vi "SerialCommunication.vi"() -> ()   [LabVIEW 2011]
uses:
  <vilib>/FPGAPlugInAG/sbRIO-9636/niLvFpga_Open_sbRIO-9636.vi
  <vilib>/rvi/interface/common/dynamic/niFpgaDynamicAddResources.vi
  <vilib>/Utility/error.llb/Error Cluster From Error Code.vi
  <vilib>/rvi/errors/niLvFpgaAdjustHostInterfaceError.vi
  <vilib>/FPGAPlugInAG/Dynamic/niLvFpga_Run_Dynamic.vi
  <vilib>/FPGAPlugInAG/Dynamic/niLvFpga_Close_Dynamic.vi
  <vilib>/rvi/interface/nirviOpenFPGA/nirviOpenFPGA.xnode
  FPGA Bitfiles/TreadmillControl_FPGATarget_Exercise2_CF30559D.lvbitx
  FPGA/FPGA.vi
  <vilib>/rvi/interface/nirviReadWriteControl/nirviReadWriteControl.xnode
  <vilib>/rvi/interface/nirviMethod/nirviMethod.xnode
  <vilib>/rvi/interface/nirviCloseFPGA/nirviCloseFPGA.xnode
  NiFpgaLv.dll
  <vilib>/rvi/interface/Simulation/niFpgaSimulationCallBeginRW.vi
  <vilib>/FPGAPlugInAG/Dynamic/niLvFpga_ReadFifo_Dynamic.vi
  <vilib>/rvi/errors/niLvFpgaMergeErrorWithErrorCode.vi
panel:
  out "Elements Remaining":u32
  out "sum":u8
  in  "baud rate":u32=2500000
  out "PacketOut":u8[](array[numeric]) format="%02x"
  in  "Vl":i16
  in  "Vr":i16
  in  "Kff":u16
  in  "Kaw":u16
  in  "Kd":u16
  in  "Ki":u16
  in  "Kp":u16
  in  "PacketType":T1(ring)
  in  "Decimation":i32
  in  "EnableLog":bool
  in  "Right":u16 format="%x"
  in  "Left":u16 format="%x"
  out "Valid":bool
  out "ReadPacket":u8[](array[numeric]) format="%x"
  in  "Write":bool
  in  "Stop":bool
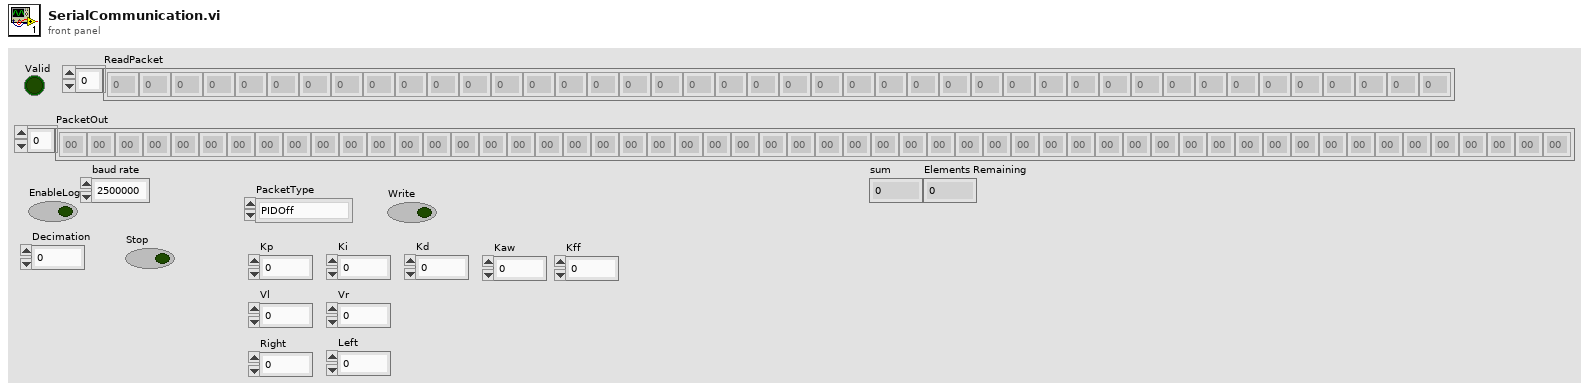
[diagram p1: front panel]
types:
  T1 = enum16{"PIDOff", "PIDOn", "PIDSetProfile", "PIDSetGains", "ThrustOpenLoop"}
  T2 = enum16{"open", "replace", "create", "open or create", "replace or create", "replace or create with confirmation"}
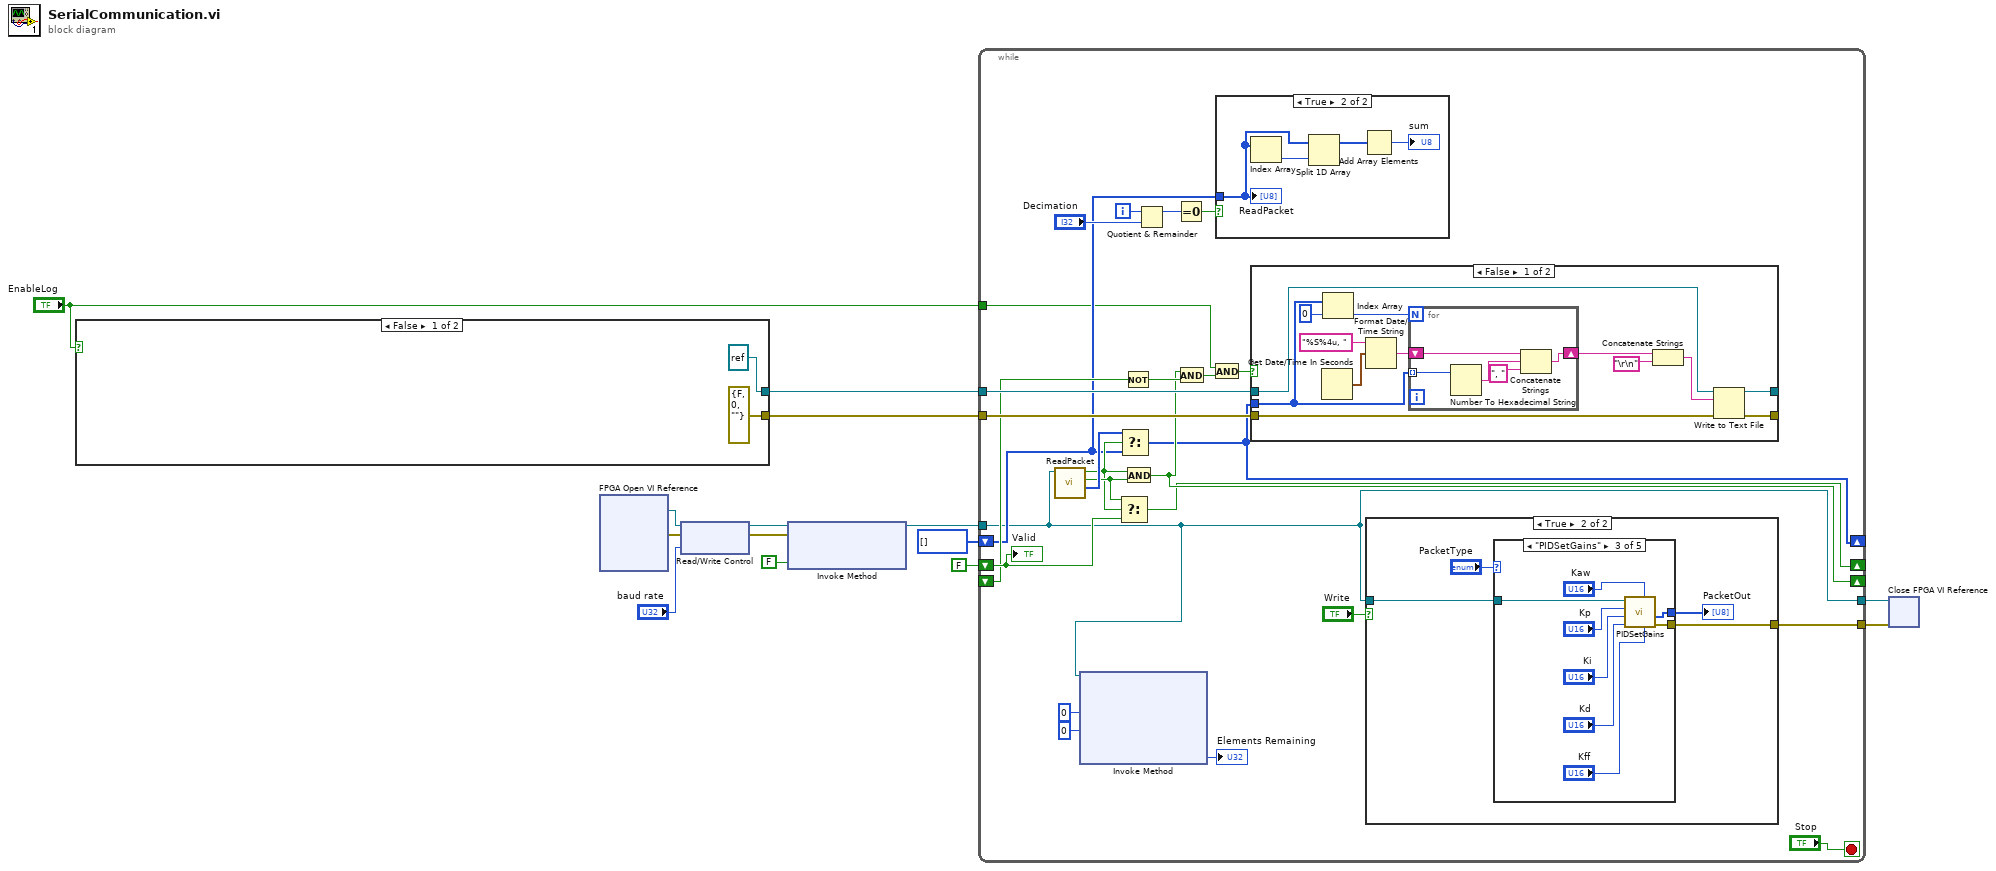
[diagram p0: block diagram]
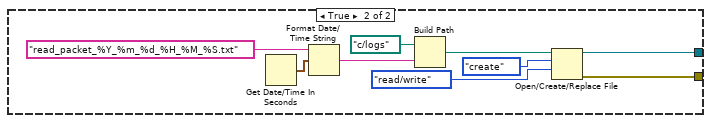
[diagram p2: hidden frame]
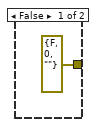
[diagram p5: hidden frame]
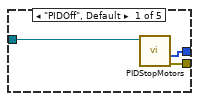
[diagram p6: hidden frame]
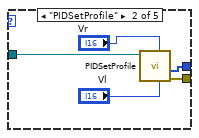
[diagram p7: hidden frame]
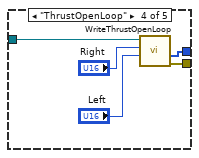
[diagram p8: hidden frame]
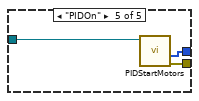
[diagram p9: hidden frame]
diagram:
  n1 = case shown="False" "EnableLog" {
    tunnel: [refnum<file> refnum ("refnum out") w18] -> w9
    tunnel: [errorcluster {"status"=FALSE, "code"=0, "source"=""} ("error out") w17] -> w8
    frame False {
    }
    frame True {
      n2 = Get Date/Time In Seconds() -> (seconds since 1Jan1904=w23:timestamp)
      n3 = Format Date/Time String(time format string (%c)="read_packet_%Y_%m_%d_%H_%M_%S.txt", seconds (now)=w23) -> (date/time string=w20:string)  [unwired: 1 in]
      n4 = Build Path(base path=path "c:/logs", name or relative path=w20) -> (appended path=w19:path)
      n5 = Open/Create/Replace File(file path (use dialog)=w19, operation (0:open)=T2."create", access (0:read/write)=enum16{"read/write", "read-only", "write-only"}."read/write") -> (refnum out=w18:refnum<file>, error out=w17:errorcluster)  [unwired: 3 in, 1 out]
    }
  }
  n6 = xnode "FPGA Open VI Reference"() -> ("FPGA VI Reference Out"=w5:refnum<k20>, "error out"=w3:errorcluster)  [unwired: 2 in]
  n7 = xnode "Read/Write Control"("FPGA VI Reference In"=w5, "error in"=w3, "baud rate"="baud rate") -> ("FPGA VI Reference Out"=w2:refnum<k20>, "error out"=w1:errorcluster)
  n8 = xnode "Invoke Method"("FPGA VI Reference In"=w2, "error in"=w1, "Wait Until Done (F)"=FALSE) -> ("FPGA VI Reference Out"=w6:refnum<k20>)  [unwired: 1 out]
  n9 = while {
    tunnel: w6 -> [w29]
    tunnel: [w50] -> w13
    tunnel: [w29] -> w12
    shift-right: [w37] -> _
    shift-left: u8[] [] ("ReadPacket") -> [w31]
    shift-right: [w36] -> _
    shift-left: FALSE ("Valid") -> [w47]
    tunnel: w9 -> [w45]
    tunnel: w8 -> [w44]
    shift-right: [w41] -> _
    shift-left: _ -> [w43]
    tunnel: "EnableLog" -> [w30]
    i -> [w35]
    stop <- "Stop" stop-if-true
    n10 = call "ReadPacket.vi"("Refnum in"=w29) -> ("ReadPacket"=w48:u8[], "Valid"=w46:bool, "Complete"=w40:bool)  [unwired: 8 in]
    n11 = xnode "Invoke Method"("FPGA VI Reference In"=w29, "Number of Elements"=u32 0, "Timeout (ms)"=0) -> ("Elements Remaining"=→"Elements Remaining":u32)  [unwired: 1 in, 3 out]
    n12 = Select(t=w46, s=w40, f=w47) -> (s? t:f=w36:bool)
    n13 = Select(t=w48, s=w40, f=w31) -> (s? t:f=w37:u8[])
    n14 = Not(x=w43) -> (.not. x?=w42:bool)
    n15 = And(x=w40, y=w46) -> (x .and. y?=w41:bool)
    n16 = Quotient & Remainder(x=w35, y="Decimation") -> (x-y*floor(x/y)=w33:i32)  [unwired: 1 out]
    n17 = Equal To 0?(x=w33) -> (x = 0?=w32:bool)
    n18 = And(x=w41, y=w42) -> (x .and. y?=w39:bool)
    n19 = And(x=w30, y=w39) -> (x .and. y?=w38:bool)
    n20 = case shown="True" w32 {
      tunnel: w31 -> [_ w55]
      frame False {
      }
      frame True {
        n21 = Index Array(array=w55) -> (element=w54:u8)  [unwired: 1 in]
        n22 = Split 1D Array(array=w55, index=w54) -> (first subarray=w53:u8[])  [unwired: 1 out]
        n23 = Add Array Elements(numeric array=w53) -> (sum=→"sum":u8)
        "ReadPacket" <- w55
      }
    }
    n24 = case shown="False" w38 {
      tunnel: w45 -> [w68 w75]
      tunnel: w44 -> [w67 w74]
      tunnel: [w66 w75] -> _
      tunnel: [w65 w74] -> _
      tunnel: w37 -> [w57 _]
      frame False {
        n25 = Get Date/Time In Seconds() -> (seconds since 1Jan1904=w58:timestamp)
        n26 = Index Array(array=w57, index=0) -> (element=w62:u8)
        n27 = Format Date/Time String(time format string (%c)="%S%4u, ", seconds (now)=w58) -> (date/time string=w61:string)  [unwired: 1 in]
        n28 = for {
          N: w62 -> [_]
          tunnel: w57 -> [w73] mode=indexing
          shift-right: [w69] -> w56
          shift-left: w61 -> [w72]
          n29 = Number To Hexadecimal String(2:w73) -> (0:w71:string)  [unwired: 1 in]
          n30 = Concatenate Strings(w72, w71, ", " ("string")) -> (w69:string)
        }
        n31 = Concatenate Strings(w56, "\r\n") -> (w59:string)
        n32 = Write to Text File(file (use dialog)=w68, text=w59, error in=w67) -> (refnum out=w66:refnum<file>, error out=w65:errorcluster)  [unwired: 1 in, 1 out]
      }
      frame True {
      }
    }
    n33 = case shown="True" "Write" {
      tunnel: w29 -> [_ w80]
      tunnel: [errorcluster {"status"=FALSE, "code"=0, "source"=""} ("error out") w79] -> w50
      frame False {
      }
      frame True {
        n34 = case shown="\"PIDSetGains\"" "PacketType" {
          tunnel: w80 -> [w83 w88 w96 w101 w104]
          tunnel: [w82 w85 w90 w100 w103] -> w79
          tunnel: [w81 w84 w89 w97 w102] -> w77
          frame "PIDOff", Default {
            n35 = call "PIDStopMotors.vi"("Refnum in"=w83) -> ("error out"=w82:errorcluster, "PacketOut"=w81:u8[])  [unwired: 9 in]
          }
          frame "PIDSetProfile" {
            n36 = call "PIDSetProfile.vi"("Refnum in"=w88, "Vr"="Vr", "Vl"="Vl") -> ("PacketOut"=w84:u8[], "error out"=w85:errorcluster)  [unwired: 5 in]
          }
          frame "PIDSetGains" {
            n37 = call "PIDSetGains.vi"("Refnum in"=w96, "Kp"="Kp", "Ki"="Ki", "Kd"="Kd", "Kaw"="Kaw", "Kff"="Kff") -> ("PacketOut"=w89:u8[], "error out"=w90:errorcluster)  [unwired: 2 in]
          }
          frame "ThrustOpenLoop" {
            n38 = call "WriteThrustOpenLoop.vi"("Left"="Left", "Right"="Right", "Refnum in"=w101) -> ("error out"=w100:errorcluster, "PacketOut"=w97:u8[])  [unwired: 7 in]
          }
          frame "PIDOn" {
            n39 = call "PIDStartMotors.vi"("Refnum in"=w104) -> ("error out"=w103:errorcluster, "PacketOut"=w102:u8[])  [unwired: 9 in]
          }
        }
        "PacketOut" <- w77
      }
    }
    "Valid" <- w47
  }
  n40 = xnode "Close FPGA VI Reference"("FPGA VI Reference In"=w12, "error in"=w13) -> ()  [unwired: 1 out]
